vi "Set Control Value.vi"(2 "error in":errorcluster, 3 "Value":variant, 4 "Controls Reference Array":refnum<vi>[](array[refnum])) -> (0 "error out":errorcluster)   [LabVIEW 2020]
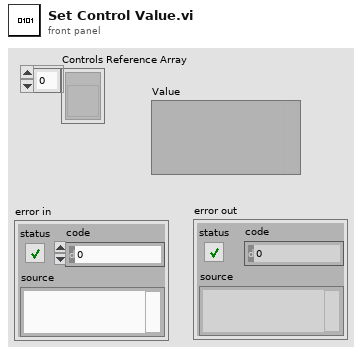
[diagram p1: front panel]
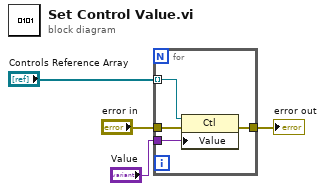
[diagram p0: block diagram]
diagram:
  n1 = for {
    tunnel: "error in" -> [w8]
    tunnel: [w7] -> w3
    tunnel: "Controls Reference Array" -> [w6] mode=indexing
    tunnel: "Value" -> [w5]
    n2 = property on="Property Node" class="Ctl"(reference=w6, error in=w8, "Value"=w5) -> (error out=w7:errorcluster)  [unwired: 1 out]
  }
  "error out" <- w3
